vi "測定キャンセルボタン.vi"() -> ()   [LabVIEW 2021]
panel:
  out "グローバル_測定キャンセルボタン":bool
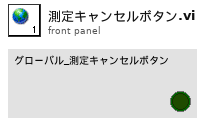
[diagram p1: front panel]
diagram:
